vi "readData.vi"(6 "error in (no error)":errorcluster, 8 "Names cluster":T1={"readSetPoint"="$R0\\?\\r\\n", "readT1"=">\\s$R100\\?\\r\\n", "readT2"=">\\s$R101\\?\\r\\n", "readT3"=">\\s$R101\\?\\r\\n", "readT4"=">\\s$R101\\?\\r\\n", "readV"=">\\s$R101\\?\\r\\n", "readI"=">\\s$R101\\?\\r\\n", "readPower"=">\\s$R153\\?\\r\\n"}, 9 "VISA resource name":refnum<visa-resource-name>) -> (0 "error out":errorcluster, 2 "Output cluster":T2 {"Power" format="%.2g"; "Voltage" format="%.2g"; "Current" format="%.2g"; "Regulator" format="%.2g"; "Extra sensor" format="%.2g"; "Cold plate" format="%.2g"; "Set point" format="%.2g"; "Main sensor" format="%.2g"}, 3 "VISA resource name out":refnum<visa-resource-name>)   [LabVIEW 2013]
uses:
  controler_custer.ctl
panel:
  # "Temeprature"
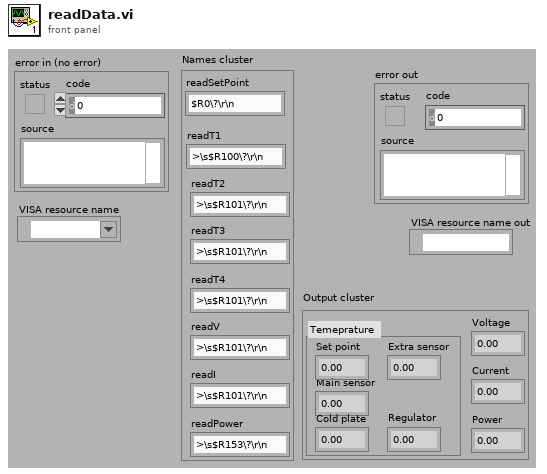
[diagram p1: front panel]
types:
  T1 = cluster{"readSetPoint":string, "readT1":string, "readT2":string, "readT3":string, "readT4":string, "readV":string, "readI":string, "readPower":string}
  T2 = typedef "controler_custer.ctl" = cluster{"Set point":dbl, "Main sensor":dbl, "Cold plate":dbl, "Extra sensor":dbl, "Regulator":dbl, "Voltage":dbl, "Current":dbl, "Power":dbl}
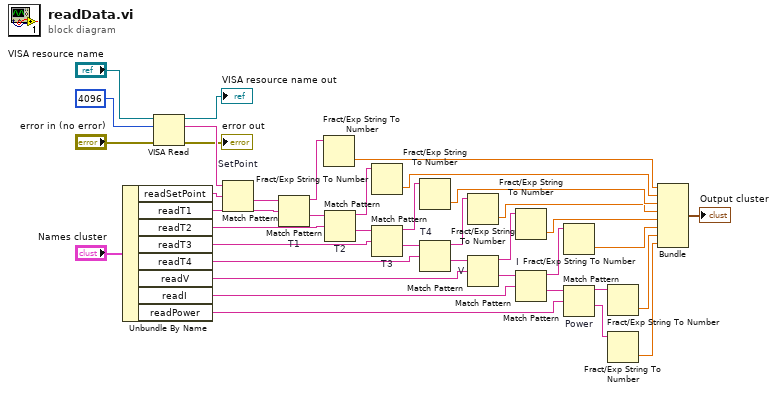
[diagram p0: block diagram]
diagram:
  n1 = Unbundle By Name("Names cluster") -> ("readSetPoint"=w10:string, "readT1"=w9:string, "readT2"=w8:string, "readT3"=w7:string, "readT4"=w6:string, "readV"=w5:string, "readI"=w4:string, "readPower"=w3:string)
  n2 = VISA Read(VISA resource name="VISA resource name", byte count=u32 4096 ("nombre d'octets"), error in (no error)="error in (no error)") -> (VISA resource name out=→"VISA resource name out":refnum<visa-resource-name>, read buffer=w24:string, error out=→"error out":errorcluster)  [unwired: 1 out]
  n3 = Match Pattern "SetPoint"(string=w24, regular expression=w10) -> (after substring=w38:string)  [unwired: 1 in, 3 out]
  n4 = Match Pattern "T1"(string=w38, regular expression=w9) -> (before substring=w36:string, after substring=w39:string)  [unwired: 1 in, 2 out]
  n5 = Fract/Exp String To Number(string=w36) -> (number=w21:dbl)  [unwired: 3 in, 1 out]
  n6 = Match Pattern "T2"(string=w39, regular expression=w8) -> (before substring=w35:string, after substring=w30:string)  [unwired: 1 in, 2 out]
  n7 = Fract/Exp String To Number(string=w35) -> (number=w20:dbl)  [unwired: 3 in, 1 out]
  n8 = Match Pattern "T3"(string=w30, regular expression=w7) -> (before substring=w29:string, after substring=w28:string)  [unwired: 1 in, 2 out]
  n9 = Fract/Exp String To Number(string=w29) -> (number=w19:dbl)  [unwired: 3 in, 1 out]
  n10 = Match Pattern "T4"(string=w28, regular expression=w6) -> (before substring=w34:string, after substring=w31:string)  [unwired: 1 in, 2 out]
  n11 = Fract/Exp String To Number(string=w34) -> (number=w18:dbl)  [unwired: 3 in, 1 out]
  n12 = Match Pattern "V"(string=w31, regular expression=w5) -> (before substring=w33:string, after substring=w37:string)  [unwired: 1 in, 2 out]
  n13 = Fract/Exp String To Number(string=w33) -> (number=w17:dbl)  [unwired: 3 in, 1 out]
  n14 = Match Pattern "I"(string=w37, regular expression=w4) -> (before substring=w32:string, after substring=w27:string)  [unwired: 1 in, 2 out]
  n15 = Fract/Exp String To Number(string=w32) -> (number=w16:dbl)  [unwired: 3 in, 1 out]
  n16 = Match Pattern "Power"(string=w27, regular expression=w3) -> (before substring=w26:string, after substring=w25:string)  [unwired: 1 in, 2 out]
  n17 = Fract/Exp String To Number(string=w26) -> (number=w15:dbl)  [unwired: 3 in, 1 out]
  n18 = Fract/Exp String To Number(string=w25) -> (number=w14:dbl)  [unwired: 3 in, 1 out]
  n19 = Bundle(w21, w20, w19, w18, w17, w16, w15, w14) -> (→"Output cluster":cluster{dbl, dbl, dbl, dbl, dbl, dbl, dbl, dbl})  [unwired: 1 in]
